vi "Autonomous Independent.vi"() -> ()   [LabVIEW 2018]
doc: "This VI is called when autonomous begins, and will automatically be terminated when autonomous ends. You can carry out timed or sensor driven robot movement independently without needing to return to the caller."
uses:
  <vilib>/Rock Robotics/WPI/DriverStation/WPI_DriverStationRobotMode2.ctl
  <vilib>/Rock Robotics/WPI/DriverStation/WPI_DriverStationDerivedRobotMode.ctl
  <vilib>/Rock Robotics/Network Tables/NT Read String.vi
  Robot Global Data.vi
panel:
  in  "Array of robot movements":T1(array[cluster])=[{"X Joystick Value"=0.39393939393939403, "Y Joystick Value"=0.0, "Delay (sec)"=1.0, "Movement Name"="turn"}, {"X Joystick Value"=-0.3737373737373737, "Y Joystick Value"=0.0, "Delay (sec)"=1.0, "Movement Name"="turn back"}] {"Y Joystick Value" scale=1.0..-1.0; "X Joystick Value" scale=-1.0..1.0}
  # "Be sure to right-click and choose Data Operations>>Make Current Value default if you want to save the array values with the VI"
  # "Test text"
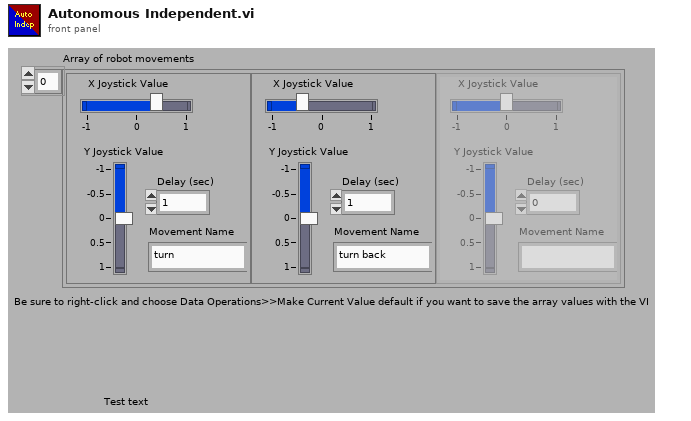
[diagram p1: front panel]
types:
  T1 = cluster{"X Joystick Value":dbl, "Y Joystick Value":dbl, "Delay (sec)":dbl, "Movement Name":string}[]
  T2 = typedef "Auton Movements.ctl" = cluster{"Drive":dbl, "TurnDegrees":dbl}
  T3 = cluster{"Encoder Counts Per Distance ":dbl, "Encoder Counts Per Distance ":dbl}
  T4 = typedef "WPI_DriverStationDerivedRobotMode.ctl" = enum16{"Init", "Execute", "Stop"}
  T5 = typedef "WPI_DriverStationRobotMode2.ctl" = enum16{"Autonomous Disabled", "Autonomous Enabled", "Teleop Disabled", "Teleop Enabled", "Disconnected", "Finish", "Test Disabled", "Test Enabled", "Emergency Stopped"}
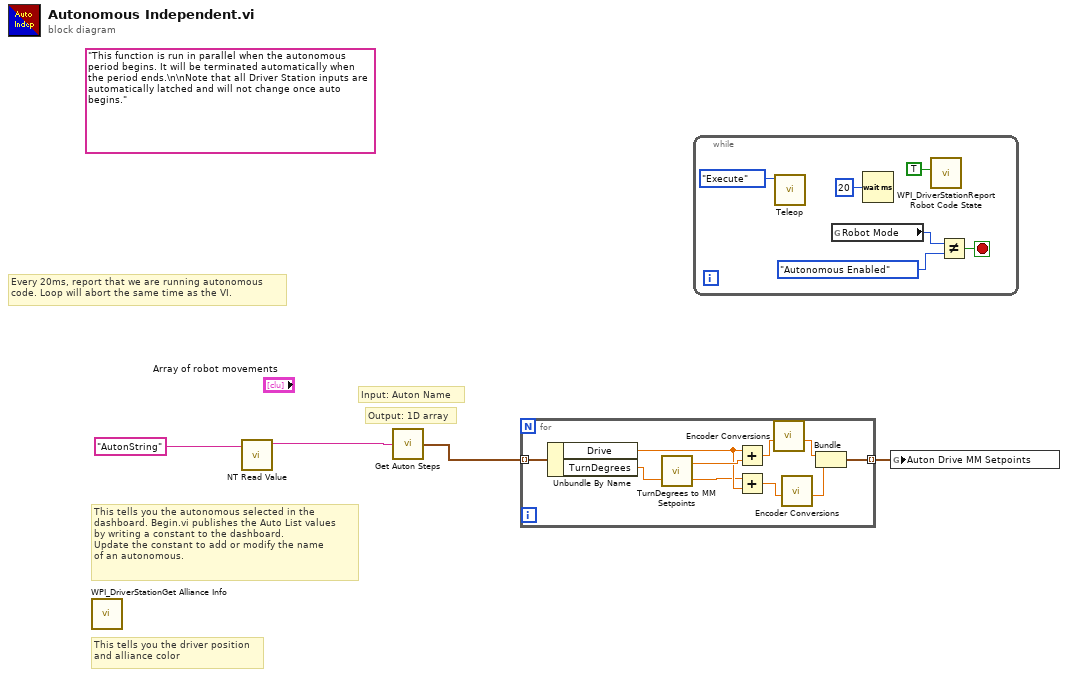
[diagram p0: block diagram]
diagram:
  (unwired) "This function is run in parallel when the autonomous period begins. It will be terminated automatically when the period ends.\n\nNote that all Driver Station inputs are automatically latched and will not change once auto begins."
  # "Input: Auton Name"
  # "Output: 1D array"
  # "This tells you the autonomous selected in the \ndashboard. Begin.vi publishes the Auto List values\nby writing a constant to the dashboard.\nUpdate the constant to add or modify the name\nof an autonomous."
  # "Every 20ms, report that we are running autonomous\ncode. Loop will abort the same time as the VI."
  # "This tells you the driver position\nand alliance color"
  n1 = call <vilib>:"WPI_DriverStationGet Alliance Info.vi"() -> ()  [unwired: 12 out]
  n2 = call-poly <vilib>:"NT Read Value.vi"("Name"="AutonString") -> ("String"=w1:string)  [unwired: 9 in, 1 out]
  n3 = call "Get Auton Steps.vi"("Name of Auton to Do"=w1) -> ("Output Movements"=w3:T2[])
  n4 = for {
    tunnel: w3 -> [w14] mode=indexing
    tunnel: [w13] -> w2 mode=indexing
    n5 = Unbundle By Name(w14) -> ("Drive"=w11:dbl, "TurnDegrees"=w9:dbl)
    n6 = call "TurnDegrees to MM Setpoints.vi"("Turn Degrees"=w9) -> ("Right MM Setpoint"=w10:dbl, "Left MM Setpoint"=w12:dbl)  [unwired: 1 in]
    n7 = Add(x=w11, y=w12) -> (x+y=w8:dbl)
    n8 = Add(x=w10, y=w11) -> (x+y=w6:dbl)
    n9 = call "Encoder Conversions.vi"("Distance (ft)"=w8) -> ("Encoder Counts Per Distance"=w7:dbl)  [unwired: 8 in, 2 out]
    n10 = call "Encoder Conversions.vi"("Distance (ft)"=w6) -> ("Encoder Counts Per Distance"=w5:dbl)  [unwired: 8 in, 2 out]
    n11 = Bundle("Encoder Counts Per Distance"=w7, "Encoder Counts Per Distance"=w5) -> (w13:T3)  [unwired: 1 in]
  }
  n12 = while {
    stop <- w17 stop-if-true
    n13 = call "Teleop.vi"("Call Context"=WPI_DriverStationDerivedRobotMode."Execute") -> ()  [unwired: 11 in]
    n14 = global read "Robot Global Data.vi" "Robot Mode"() -> (w19:T5)
    n15 = Wait (ms)(milliseconds to wait=u32 20) -> ()  [unwired: 1 out]
    n16 = call <vilib>:"WPI_DriverStationReport Robot Code State.vi"("Autonomous"=TRUE) -> ()  [unwired: 10 in, 1 out]
    n17 = Not Equal?(x=w19, y=WPI_DriverStationRobotMode2."Autonomous Enabled" ("Robot Mode")) -> (x != y?=w17:bool)
  }
  n18 = global write "Robot Global Data.vi" "Auton Drive MM Setpoints"(w2) -> ()
